vi "Amp & Freq Estimate.vi"(2 "Size of FFT":i32=1024 min=0 step=1, 3 "window":T1(ring)=enum."7 Term B-Harris", 4 "Part of Power Spectrum":dbl[](array[numeric]) format="%0.12f") -> (0 "Exact Freq Index":dbl format="%0.6f", 1 "Exact Amplitude (Vrms)":dbl format="%0.6e")   [LabVIEW 2018, in "NI_AALPro.lvlib"]
doc: "Finds the highest peak in the spectrum and uses ADJACENT frequencies to determine where to search for the exact peak and peak location."
uses:
  NI_AALPro.lvlib
panel:
  in  "Freq. Resolution":dbl=1e-08 format="%0.2e"
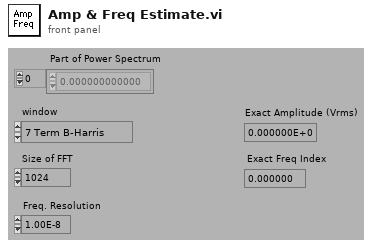
[diagram p1: front panel]
types:
  T1 = enum32{"None ", "Hanning", "Hamming", "Blackman-Harris", "Exact Blackman", "Blackman", "Flat Top", "4 Term B-Harris ", "7 Term B-Harris"}
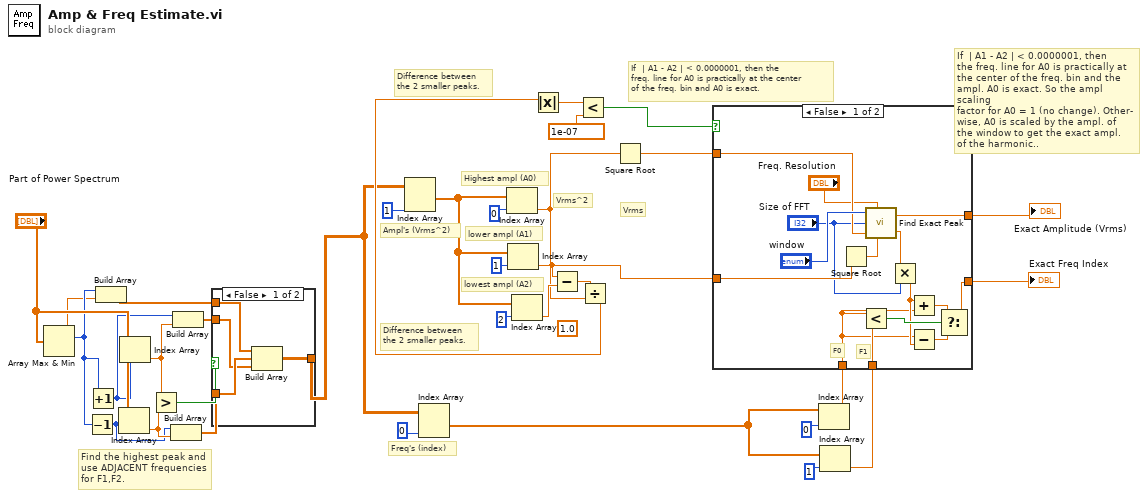
[diagram p0: block diagram]
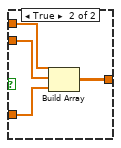
[diagram p3: hidden frame]
diagram:
  (unwired) 1.0
  # "Find the highest peak and\nuse ADJACENT frequencies\nfor F1,F2."
  # "If  | A1 - A2 | < 0.0000001, then \nthe freq. line for A0 is practically at \nthe center of the freq. bin and the \nampl. A0 is exact. So the ampl scaling \nfactor for A0 = 1 (no change). Other-\nwise, A0 is scaled by the ampl. of\nthe window to get the exact ampl.\nof the harmonic.."
  # "If  | A1 - A2 | < 0.0000001, then the\nfreq. line for A0 is practically at the center\nof the freq. bin and A0 is exact."
  # "Difference between\nthe 2 smaller peaks."
  # "Difference between\nthe 2 smaller peaks."
  # "Vrms"
  # "Vrms^2"
  # "lowest ampl (A2)"
  # "lower ampl (A1)"
  # "Highest ampl (A0)"
  # "Ampl's (Vrms^2)"
  # "Freq's (index)"
  n1 = Array Max & Min(array="Part of Power Spectrum") -> (max value=w13:dbl, max index (indices)=w14:i32)  [unwired: 2 out]
  n2 = Decrement(x=w14) -> (x-1=w17:i32)
  n3 = Increment(x=w14) -> (x+1=w19:i32)
  n4 = Build Array(w14, w13) -> (w12:dbl[])
  n5 = Index Array(array="Part of Power Spectrum", index=w17) -> (element=w18:dbl)
  n6 = Index Array(array="Part of Power Spectrum", index=w19) -> (element=w20:dbl)
  n7 = Greater?(x=w20, y=w18) -> (0:w21:bool)
  n8 = Build Array(w17, w18) -> (w16:dbl[])
  n9 = Build Array(w19, w20) -> (w15:dbl[])
  n10 = case shown="False" w21 {
    tunnel: w16 -> [w36 w40]
    tunnel: w15 -> [w35 w42]
    tunnel: w12 -> [w38 w41]
    tunnel: [w37 w39] -> w11
    frame False {
      n11 = Build Array(w38, w36, w35) -> (w37:dbl[][])
    }
    frame True {
      n12 = Build Array(w41, w42, w40) -> (w39:dbl[][])
    }
  }
  n13 = Index Array(array=w11, index (col)=1) -> (element=w29:dbl[])  [unwired: 1 in]
  n14 = Index Array(array=w11, index (col)=0) -> (element=w3:dbl[])  [unwired: 1 in]
  n15 = Index Array(array=w29, index=0) -> (element=w23:dbl)
  n16 = Index Array(array=w29, index=1) -> (element=w7:dbl)
  n17 = Index Array(array=w29, index=2) -> (element=w28:dbl)
  n18 = Subtract(x=w7, y=w28) -> (x-y=w26:dbl)
  n19 = Divide(x=w26, y=w23) -> (x/y=w24:dbl)
  n20 = Absolute Value(x=w24) -> (abs(x)=w25:dbl)
  n21 = Less?(x=w25, y=1e-07) -> (x < y?=w9:bool)
  n22 = Square Root(x=w23) -> (sqrt(x)=w8:dbl)
  n23 = Index Array(array=w3, index=0) -> (element=w6:dbl)
  n24 = Index Array(array=w3, index=1) -> (element=w4:dbl)
  n25 = case shown="False" w9 {
    tunnel: w8 -> [w55 w58]
    tunnel: w7 -> [w54 _]
    tunnel: [w43 w59] -> w2
    tunnel: w6 -> [w45 w59]
    tunnel: [w51 w58] -> w1
    tunnel: w4 -> [w49 _]
    frame False {
      # "F1"
      # "F0"
      n26 = Square Root(x=w54) -> (sqrt(x)=w57:dbl)
      n27 = Less?(x=w45, y=w49) -> (x < y?=w48:bool)
      n28 = call "Find Exact Peak.vi"("window"="window", "Freq. Resolution"="Freq. Resolution", "Size of FFT (N)"="Size of FFT", "A0"=w55, "A1"=w57) -> ("A exact"=w51:dbl, "f exact"=w53:dbl)
      n29 = Multiply(x=w53, y="Size of FFT") -> (x*y=w47:dbl)
      n30 = Add(x=w47, y=w45) -> (x+y=w46:dbl)
      n31 = Subtract(x=w45, y=w47) -> (x-y=w44:dbl)
      n32 = Select(t=w46, s=w48, f=w44) -> (s? t:f=w43:dbl)
    }
    frame True {
    }
  }
  "Exact Amplitude (Vrms)" <- w1
  "Exact Freq Index" <- w2
